vi "Read Persistent Layers.vi"(11 "Base Spawn in":refnum<class "Base Spawn.lvclass">) -> (2 "Persistent Layers":refnum<class "Actor.lvclass">[](array[class]))   [LabVIEW 2025, in "jettl.lvlib" / "Spawn.lvlib" / "Base Spawn.lvclass"]
uses:
  Base Spawn.lvclass
  Base Spawn.lvclass/Base Spawn.ctl
  Actor/Actor.lvclass
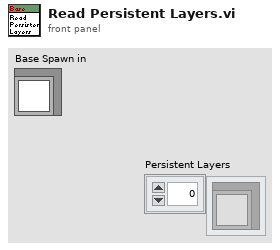
[diagram p1: front panel]
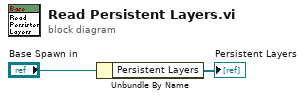
[diagram p0: block diagram]
diagram:
  n1 = Unbundle By Name("Base Spawn in") -> ("Persistent Layers"=→"Persistent Layers":refnum<class "Actor.lvclass">[])
